vi "Init_Arduino.vi"(2 "error in (no error)":errorcluster, 3 "Velocidad de Conexion":enum16{"115200", "9600"}(ring), 4 "VISA Refnum in":refnum<visa-resource-name>) -> (0 "error out":errorcluster, 1 "VISA Refnum out":refnum<visa-resource-name>)   [LabVIEW 2014]
uses:
  <vilib>/Instr/_visa.llb/VISA Find Search Mode.ctl
  <vilib>/Instr/_visa.llb/VISA Configure Serial Port (Instr).vi
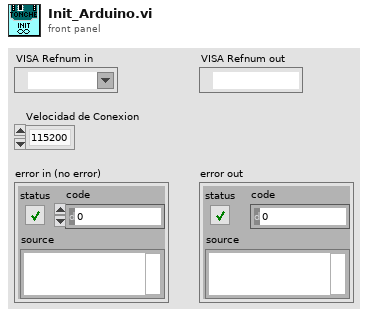
[diagram p1: front panel]
types:
  T1 = typedef "VISA Find Search Mode.ctl" = u32
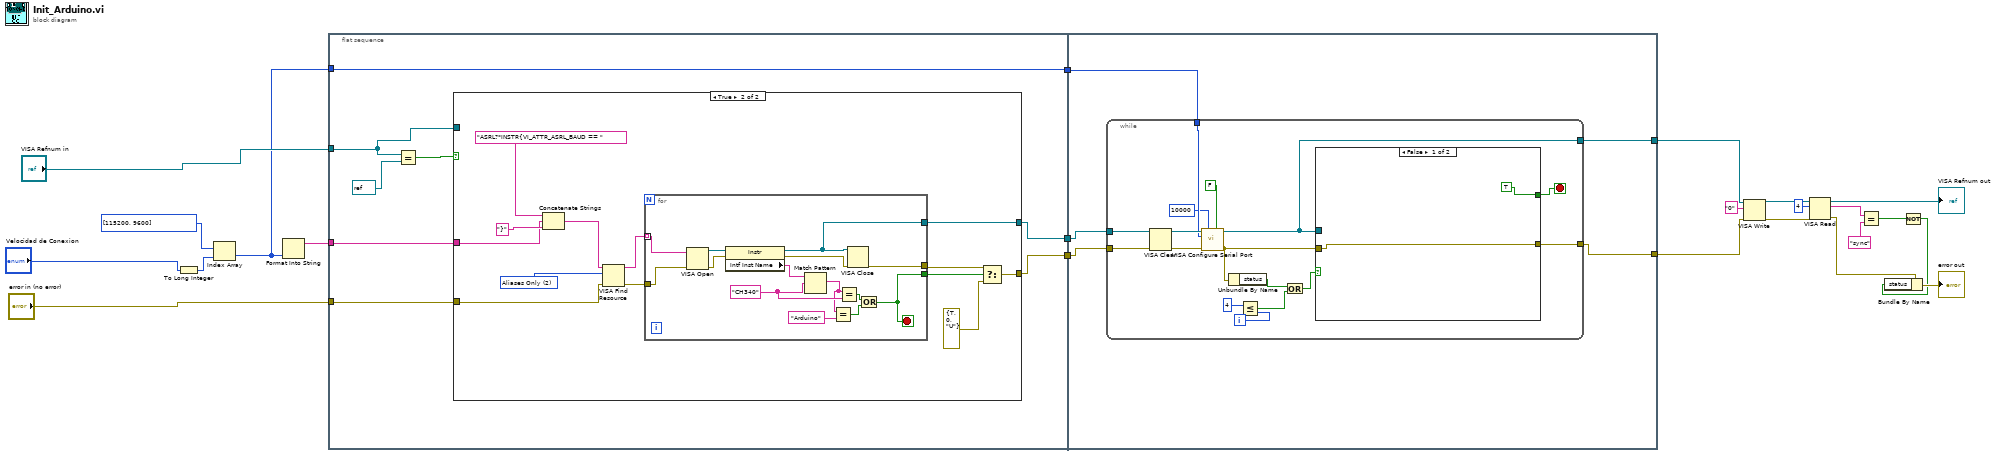
[diagram p0: block diagram]
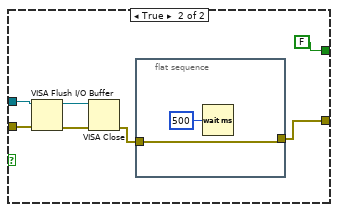
[diagram p3: hidden frame]
diagram:
  n1 = To Long Integer(number="Velocidad de Conexion") -> (32bit integer=w3:i32)
  n2 = Index Array(array=i32[] [115200, 9600], index=w3) -> (element=w17:i32)
  n3 = Format Into String(w17) -> (resulting string=w5:string)  [unwired: 3 in, 1 out]
  n4 = flat-sequence {
    tunnel: "VISA Refnum in" -> [w29]
    tunnel: "error in (no error)" -> [w28]
    tunnel: w5 -> [w27]
    tunnel: w17 -> [w24]
    tunnel: [w26] -> w23
    tunnel: [w25] -> w22
    tunnel: [w24] -> w21
    tunnel: w23 -> [w63]
    tunnel: w22 -> [w64]
    tunnel: w21 -> [w65]
    tunnel: [w62] -> w18
    tunnel: [w61] -> w19
    frame #0 {
      n5 = Equal?(x=w29, y=refnum<visa-resource-name> refnum ("VISA resource name 2")) -> (x = y?=w30:bool)
      n6 = case shown="True" w30 {
        tunnel: [w33 w37] -> w25
        tunnel: w29 -> [w32 _]
        tunnel: w28 -> [w33 w36]
        tunnel: [w32 w35] -> w26
        tunnel: w27 -> [_ w34]
        frame False {
        }
        frame True {
          w46 = T1 2 items=["Canonical Names Only"=0, "Aliases Only"=2, "Include Matching Aliases"=3, "Include All Aliases"=4] ("Search Mode")
          n7 = Concatenate Strings("ASRL?*INSTR{VI_ATTR_ASRL_BAUD == " ("string"), w34, "}" ("string")) -> (w41:string)
          n8 = VISA Find Resource(8:w36, 10:w46, 11:w41) -> (0:w44:errorcluster, 3:w45:string[])  [unwired: 1 out]
          n9 = for {
            tunnel: w45 -> [w59] mode=indexing
            tunnel: w44 -> [w60]
            tunnel: [w55] -> w35
            tunnel: [w53] -> w40
            tunnel: [w52] -> w38
            stop <- w52 stop-if-true
            w50 = "CH340" ("regular expression")
            n10 = VISA Open(error in (no error)=w60, VISA resource name=w59) -> (VISA resource name=w58:refnum<visa-resource-name>, error out=w57:errorcluster)  [unwired: 3 in]
            n11 = property class="Instr"(reference=w58, error in=w57) -> (reference out=w55:refnum<visa-resource-name>, error out=w54:errorcluster, "Intf Inst Name"=w56:string)
            n12 = Match Pattern(string=w56, regular expression=w50) -> (match substring=w48:string)  [unwired: 1 in, 3 out]
            n13 = Equal?(x=w48, y="Arduino") -> (x = y?=w49:bool)
            n14 = Equal?(x=w48, y=w50) -> (x = y?=w51:bool)
            n15 = VISA Close(VISA resource name=w55, error in (no error)=w54) -> (error out=w53:errorcluster)
            n16 = Or(x=w51, y=w49) -> (x .or. y?=w52:bool)
          }
          n17 = Select(t=w40, s=w38, f=errorcluster {"status"=TRUE, "code"=0, "source"="U"} ("error out")) -> (s? t:f=w37:errorcluster)
        }
      }
    }
    frame #1 {
      n18 = while {
        tunnel: w65 -> [w79]
        tunnel: w63 -> [w76]
        tunnel: w64 -> [w75]
        tunnel: [w67] -> w61
        tunnel: [w66] -> w62
        i -> [w73]
        stop <- w68 stop-if-true
        n19 = VISA Clear(VISA resource name=w76, error in (no error)=w75) -> (VISA resource name out=w81:refnum<visa-resource-name>, error out=w80:errorcluster)
        n20 = call-poly "VISA Configure Serial Port"("VISA resource name"=w81, "timeout (10sec)"=u32 10000, "Enable Termination\nChar (T)"=FALSE ("Enable Termination\nChar (T)"), "baud rate (9600)"=w79, "error in (no error)"=w80) -> ("VISA resource name out"=w66:refnum<visa-resource-name>, "error out"=w69:errorcluster)  [unwired: 9 in]
        n21 = Unbundle By Name(w69) -> ("status"=w74:bool)
        n22 = Less Or Equal?(x=4, y=w73) -> (x <= y?=w71:bool)
        n23 = Or(x=w74, y=w71) -> (x .or. y?=w70:bool)
        n24 = case shown="False" w70 {
          tunnel: w69 -> [w82 w90]
          tunnel: w66 -> [_ w89]
          tunnel: [TRUE FALSE] -> w68
          tunnel: [w82 w84] -> w67
          frame False {
          }
          frame True {
            n25 = VISA Flush I/O Buffer(VISA resource name=w89, error in (no error)=w90) -> (VISA resource name out=w87:refnum<visa-resource-name>, error out=w88:errorcluster)  [unwired: 1 in]
            n26 = VISA Close(VISA resource name=w87, error in (no error)=w88) -> (error out=w85:errorcluster)
            n27 = flat-sequence {
              tunnel: [w91] -> w84
              tunnel: w85 -> [w91]
              frame #0 {
                n28 = Wait (ms)(milliseconds to wait=u32 500) -> ()  [unwired: 1 out]
              }
            }
          }
        }
      }
    }
  }
  n29 = VISA Write(VISA resource name=w18, write buffer="0", error in (no error)=w19) -> (VISA resource name out=w7:refnum<visa-resource-name>, error out=w8:errorcluster)  [unwired: 1 out]
  n30 = VISA Read(VISA resource name=w7, byte count=u32 4, error in (no error)=w8) -> (VISA resource name out=→"VISA Refnum out":refnum<visa-resource-name>, read buffer=w9:string, error out=w11:errorcluster)  [unwired: 1 out]
  n31 = Equal?(x=w9, y="sync") -> (x = y?=w12:bool)
  n32 = Not(x=w12) -> (.not. x?=w13:bool)
  n33 = Bundle By Name(cluster=w11, "status"=w13) -> (→"error out":errorcluster)
